vi "CSV_Writer.vi"(0 "Array In":dbl[][](array[numeric]) caption="2D-Daten" format="%0.2f", 1 "ProFile In":path caption="Dateipfad (Dialog, wenn leer)") -> ()   [LabVIEW 2016]
uses:
  <vilib>/Utility/file.llb/Write To Spreadsheet File (DBL).vi
panel:
  out "ProFile Out":path caption="Neuer Dateipfad"
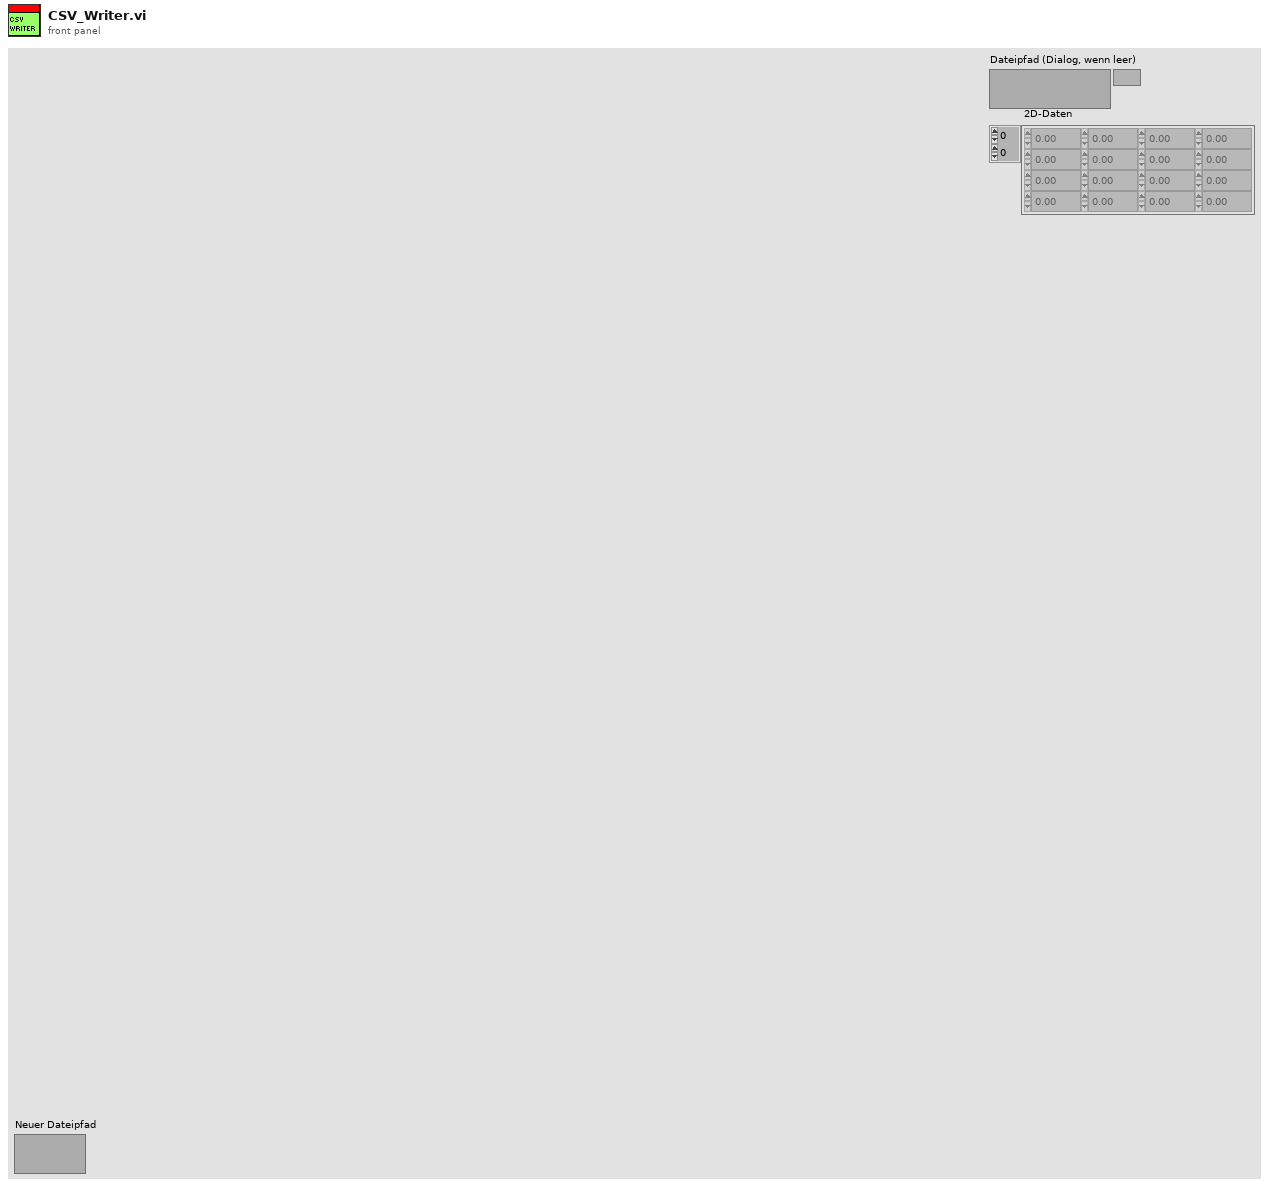
[diagram p1: front panel]
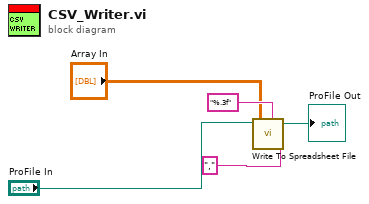
[diagram p0: block diagram]
diagram:
  n1 = call-poly <vilib>:"Write To Spreadsheet File.vi"("delimiter (\\t)"="," ("delimiter (\\t)"), "format (%.3f)"="%.3f", "2D data"="Array In", "file path (dialog if empty)"="ProFile In") -> ("new file path (Not A Path if cancelled)"=→"ProFile Out":path)  [unwired: 4 in]
